vi "MFC_SP-Read.vi"() -> ()   [LabVIEW 2014]
uses:
  <vilib>/rvi/Emulation/niFpgaGetClockAttributes.vi
  <vilib>/rvi/Emulation/niFpgaSctlEmulationGetInTimedLoop.vi
  <vilib>/rvi/Emulation/niFpgaEmulationReportErrorSimple.vi
  <vilib>/rvi/Emulation/niFpgaCriticalErrorInLSC.vi
panel:
  in  "MFC SPs":u8[](array[numeric])
  out "MFC CO-1":u8[](array[numeric])
  out "MFC HC-1":u8[](array[numeric])
  out "MFC AIR-1":u8[](array[numeric])
  out "MFC NO":u8[](array[numeric])
  out "MFC Air-B":u8[](array[numeric])
  out "MFC Array Out":u8[](array[numeric])=[65, 48, 48, 48, 48, 48, 13, 66, 48, 48, 48, 48, 48, 13, 67, 48, 48, 48, 48, 48, 13, 68, 48, 48, 48, 48, 48, 13, 73, 48, 48, 48, 48, 48, 13, 74, 48, 48, 48, 48, 48, 13, 75, 48, 48, 48, 48, 48, 13, 77, 48, 48, 48, 48, 48, 13, 0, 0, 0, 0]
  out "MFC Array In":fxp<+/-,30,9>[](array[numeric])
  out "MFC HC-B":u8[](array[numeric])
  out "MFC Air-2":u8[](array[numeric])
  out "MFC HC-2":u8[](array[numeric])
  out "MFC Error No.":u8
  out "MFC N2":u8[](array[numeric])
  out "MFC O2":u8[](array[numeric])
  out "MFC N2-2":u8[](array[numeric])
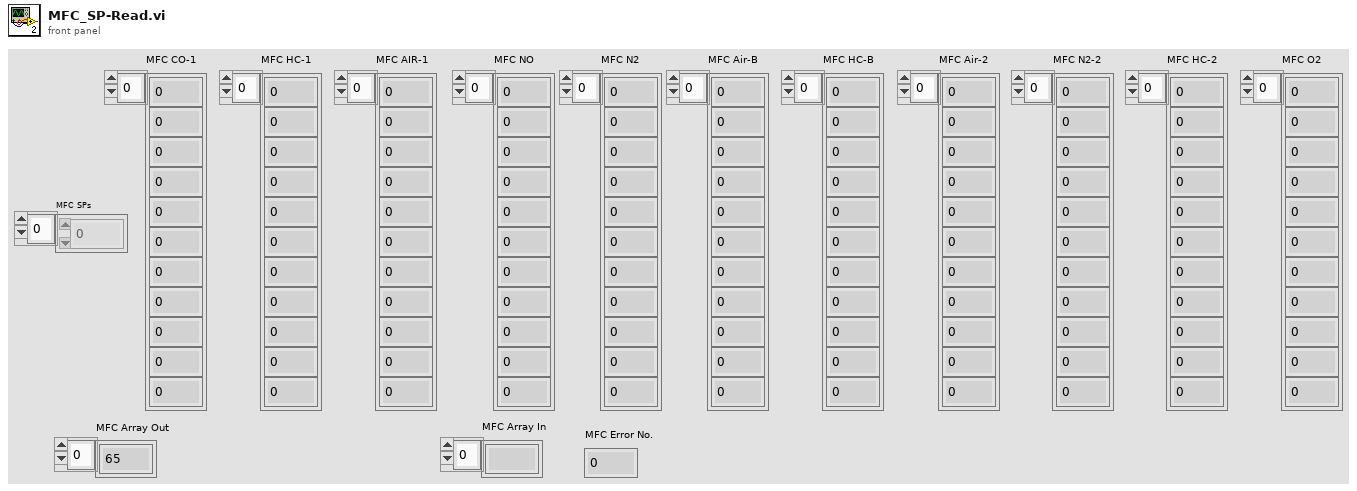
[diagram p1: front panel]
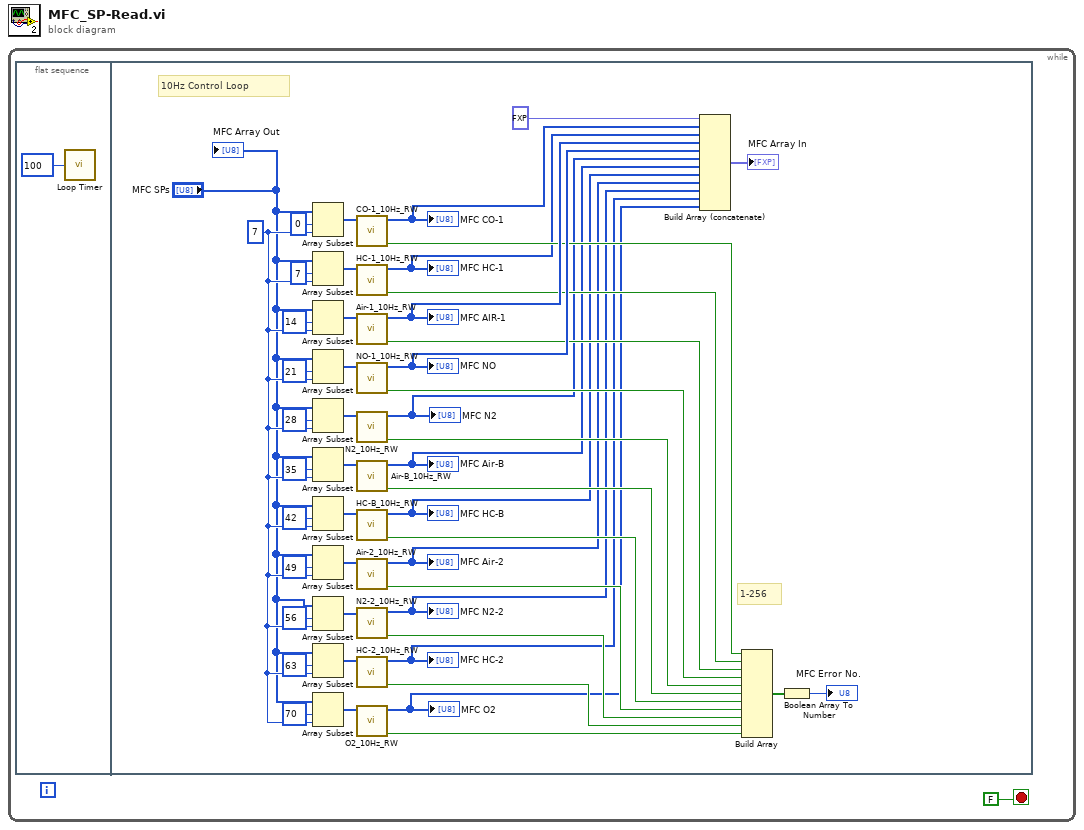
[diagram p0: block diagram]
diagram:
  n1 = while {
    stop <- FALSE stop-if-true
    n2 = flat-sequence {
      frame #0 {
        n3 = call "Loop Timer"("Count(mSec)"=u32 100) -> ()  [unwired: 1 out]
      }
      frame #1 {
        w25 = 7 ("length")
        # "1-256"
        # "10Hz Control Loop"
        n4 = Array Subset(array="MFC SPs", index=0, length=w25) -> (w42:u8[])
        n5 = Array Subset(array="MFC SPs", index=7, length=w25) -> (w41:u8[])
        n6 = Array Subset(array="MFC SPs", index=14, length=w25) -> (w40:u8[])
        n7 = Array Subset(array="MFC SPs", index=21, length=w25) -> (w39:u8[])
        n8 = Array Subset(array="MFC SPs", index=28, length=w25) -> (w29:u8[])
        n9 = Array Subset(array="MFC SPs", index=35, length=w25) -> (w38:u8[])
        n10 = Array Subset(array="MFC SPs", index=42, length=w25) -> (w37:u8[])
        n11 = Array Subset(array="MFC SPs", index=49, length=w25) -> (w36:u8[])
        n12 = Array Subset(array="MFC SPs", index=56, length=w25) -> (w27:u8[])
        n13 = Array Subset(array="MFC SPs", index=63, length=w25) -> (w35:u8[])
        n14 = Array Subset(array="MFC SPs", index=70, length=w25) -> (w24:u8[])
        n15 = call "CO-1_10Hz_RW.vi"("Byte Array"=w42) -> ("Fault"=w23:bool, "MFC out"=w7:u8[])  [unwired: 9 in]
        "MFC CO-1" <- w7
        n16 = call "HC-1_10Hz_RW.vi"("Byte Array"=w41) -> ("Fault"=w22:bool, "MFC out"=w8:u8[])  [unwired: 9 in]
        "MFC HC-1" <- w8
        n17 = call "Air-1_10Hz_RW.vi"("Byte Array"=w40) -> ("Fault"=w21:bool, "MFC out"=w34:u8[])  [unwired: 9 in]
        "MFC AIR-1" <- w34
        n18 = call "NO-1_10Hz_RW.vi"("Byte Array"=w39) -> ("Fault"=w20:bool, "MFC out"=w33:u8[])  [unwired: 9 in]
        "MFC NO" <- w33
        n19 = call "N2_10Hz_RW.vi"("Byte Array"=w29) -> ("Fault"=w19:bool, "MFC out"=w5:u8[])  [unwired: 9 in]
        "MFC N2" <- w5
        n20 = call "Air-B_10Hz_RW.vi"("Byte Array"=w38) -> ("Fault"=w18:bool, "MFC out"=w12:u8[])  [unwired: 9 in]
        "MFC Air-B" <- w12
        n21 = call "HC-B_10Hz_RW.vi"("Byte Array"=w37) -> ("Fault"=w17:bool, "MFC out"=w11:u8[])  [unwired: 9 in]
        "MFC HC-B" <- w11
        n22 = call "Air-2_10Hz_RW.vi"("Byte Array"=w36) -> ("Fault"=w16:bool, "MFC out"=w10:u8[])  [unwired: 9 in]
        "MFC Air-2" <- w10
        n23 = call "N2-2_10Hz_RW.vi"("Byte Array"=w27) -> ("Fault"=w15:bool, "MFC out"=w4:u8[])  [unwired: 9 in]
        "MFC N2-2" <- w4
        n24 = call "HC-2_10Hz_RW.vi"("Byte Array"=w35) -> ("Fault"=w14:bool, "MFC out"=w9:u8[])  [unwired: 9 in]
        "MFC HC-2" <- w9
        n25 = call "O2_10Hz_RW.vi"("Byte Array"=w24) -> ("Fault"=w13:bool, "MFC out"=w6:u8[])  [unwired: 9 in]
        "MFC O2" <- w6
        n26 = Build Array (concatenate)(fxp<+/-,26,5> 0.0 ("Pressure_Tank"), w7, w8, w34, w33, w5, w12, w11, w10, w4, w9, w6) -> (→"MFC Array In":fxp<+/-,30,9>[])
        n27 = Build Array(w23, w22, w21, w20, w19, w18, w17, w16, w15, w14, w13) -> (w44:bool[])
        n28 = Boolean Array To Number(Boolean array=w44) -> (number=→"MFC Error No.":u16)
        "MFC Array Out" <- "MFC SPs"
      }
    }
  }
